vi "fit mag to ellipse.vi"(9 "T":dbl, 10 "t0":dbl, 11 "mag no drive":T1[](array[typedef])) -> (1 "fitter error":bool, 2 "fit magnetic field":T1[](array[typedef]), 3 "fit parameters":cluster{"a":dbl, "b":dbl, "theta":dbl, "b0":dbl})   [LabVIEW 2017]
uses:
  typedefs/reading.ctl
  typedefs/readingType.ctl
  <vilib>/gmath/NumericalOptimization/Nonlinear Curve Fit LM.vi
  <vilib>/gmath/NI_Gmath.lvlib
panel:
  out "phi":dbl[](array[numeric])
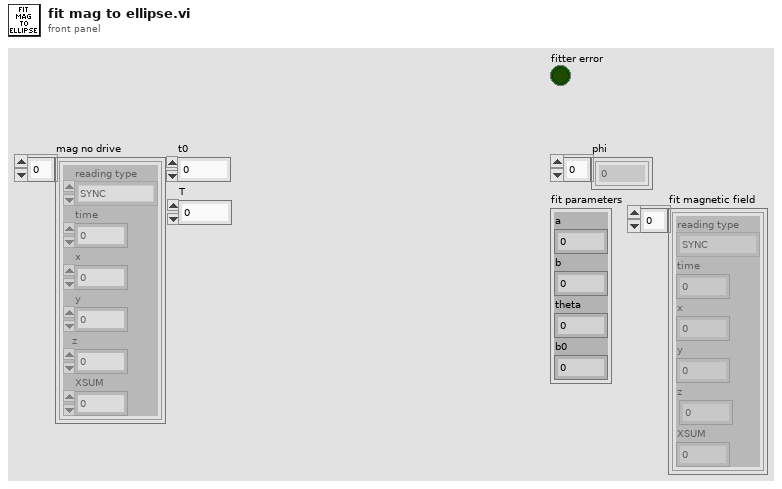
[diagram p1: front panel]
types:
  T1 = typedef "reading.ctl" = cluster{"reading type":T2, "time":fxp<+,48,48>, "x":sgl, "y":sgl, "z":sgl, "XSUM":u8}
  T2 = typedef "readingType.ctl" = enum8{"SYNC", "DETVAL", "COILI", "MAGVEC", "ACCVEC"}
  T3 = cluster{"best fit parameters[0]":dbl, "best fit parameters[1]":dbl, "best fit parameters[2]":dbl, "best fit parameters[3]":dbl}
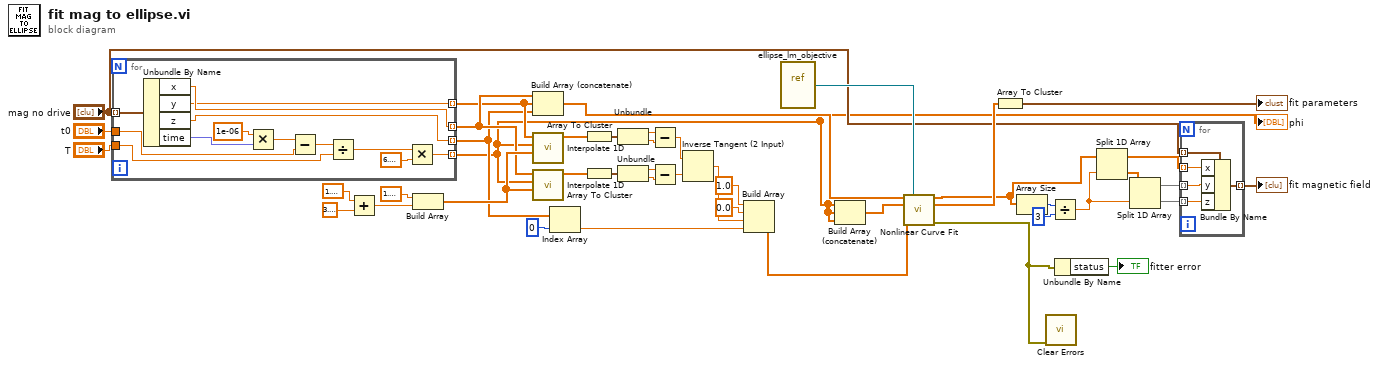
[diagram p0: block diagram]
diagram:
  n1 = for {
    tunnel: "mag no drive" -> [w57] mode=indexing
    tunnel: "T" -> [w54]
    tunnel: "t0" -> [w56]
    tunnel: [w48] -> w4 mode=indexing
    tunnel: [w47] -> w22 mode=indexing
    tunnel: [w46] -> w21 mode=indexing
    tunnel: [w45] -> w20 mode=indexing
    n2 = Unbundle By Name(w57) -> ("x"=w47:sgl, "y"=w46:sgl, "z"=w45:sgl, "time"=w51:fxp<+,48,48>)
    n3 = Multiply(x=1e-06, y=w51) -> (x*y=w50:dbl)
    n4 = Subtract(x=w50, y=w56) -> (x-y=w55:dbl)
    n5 = Divide(x=w55, y=w54) -> (x/y=w53:dbl)
    n6 = Multiply(x=w53, y=6.283185307179586) -> (x*y=w48:dbl)
  }
  "phi" <- w4
  n7 = Add(x=1.5707963267948966, y=3.141592653589793) -> (x+y=w39:dbl)
  n8 = Build Array(1.5707963267948966, w39) -> (w38:dbl[])
  n9 = Build Array (concatenate)(w22, w21, w20) -> (w19:sgl[])
  n10 = call <vilib>:"Interpolate 1D.vi"("xi"=w38, "X"=w4, "Y"=w21) -> ("yi"=w36:dbl[])  [unwired: 6 in, 2 out]
  n11 = call <vilib>:"Interpolate 1D.vi"("xi"=w38, "X"=w4, "Y"=w22) -> ("yi"=w37:dbl[])  [unwired: 6 in, 2 out]
  n12 = Index Array(array=w20, index=0) -> (element=w23:sgl)
  n13 = Array To Cluster(array=w36) -> (cluster=w34:cluster{"yi[0]":dbl, "yi[1]":dbl})
  n14 = Array To Cluster(array=w37) -> (cluster=w35:cluster{"yi[0]":dbl, "yi[1]":dbl})
  n15 = Unbundle(w34) -> ("yi[0]"=w31:dbl, "yi[1]"=w30:dbl)
  n16 = Unbundle(w35) -> ("yi[0]"=w33:dbl, "yi[1]"=w32:dbl)
  n17 = Subtract(x=w31, y=w30) -> (x-y=w29:dbl)
  n18 = Subtract(x=w33, y=w32) -> (x-y=w28:dbl)
  n19 = Inverse Tangent (2 Input)(1:w28, 2:w29) -> (0:w24:dbl)
  n20 = Build Array(1.0 ("element"), 0.0 ("element"), w24, w23) -> (w18:dbl[])
  n21 = vi-ref "ellipse_lm_objective.vi"() -> (w16:refnum<vi>)
  n22 = Build Array (concatenate)(w4, w4, w4) -> (w5:dbl[])
  n23 = call-poly <vilib>:"Nonlinear Curve Fit.vi"("Y"=w19, "f(x,a)"=w16, "X"=w5, "initial parameters"=w18) -> ("best nonlinear fit"=w3:dbl[], "best fit parameters"=w13:dbl[], "error out"=w7:errorcluster)  [unwired: 6 in, 3 out]
  n24 = Array To Cluster(array=w13) -> (cluster=→"fit parameters":T3)
  n25 = Array Size(array=w3) -> (size(s)=w15:i32)
  n26 = call <vilib>:"Clear Errors.vi"("error in (no error)"=w7) -> ()  [unwired: 5 in, 2 out]
  n27 = Divide(x=w15, y=3) -> (x/y=w1:dbl)
  n28 = Unbundle By Name(w7) -> ("status"=→"fitter error":bool)
  n29 = Split 1D Array(array=w3, index=w1) -> (first subarray=w12:dbl[], second subarray=w2:dbl[])
  n30 = Split 1D Array(array=w2, index=w1) -> (first subarray=w11:dbl[], second subarray=w10:dbl[])
  n31 = for {
    tunnel: w12 -> [w61] mode=indexing
    tunnel: w11 -> [w60] mode=indexing
    tunnel: w10 -> [w59] mode=indexing
    tunnel: "mag no drive" -> [w62] mode=indexing
    tunnel: [w58] -> w8 mode=indexing
    n32 = Bundle By Name(cluster=w62, "x"=w61, "y"=w60, "z"=w59) -> (w58:T1)
  }
  "fit magnetic field" <- w8
